vi "Set DO Status - Single.vi"(0 "reference in":refnum<class "DO.lvclass">, 2 "DO Channel Number (Zero Based)":i32, 4 "DO Status to Set":bool, 5 "error in (no error)":errorcluster) -> (14 "reference out":refnum<class "DO.lvclass">, 16 "DO Channel Number (Zero Based) OUT":i32, 19 "error out":errorcluster)   [LabVIEW 2017, in "DO.lvclass"]
uses:
  DO.lvclass
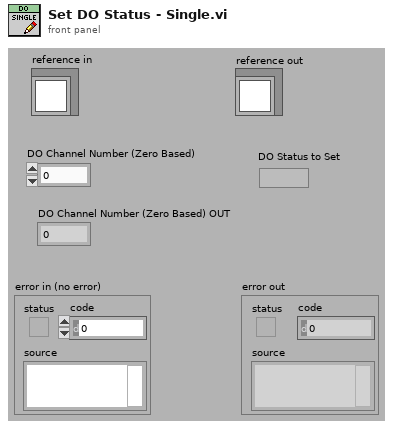
[diagram p1: front panel]
types:
  T1 = typedef "DO.lvclass/ObjectAttributes.ctl" = cluster{"DO Task":refnum<k21>, "DO Module Names (NI-Max Name)":string[], "Number of Channels Per DO Module":i32[], "DO Status":bool[], "Number of DO Modules":u32, "DO Status to Set":bool[], "DO On/Off Status":bool, "DO VI Reference":refnum<vi>, "Number of Total DO Channels":u32}
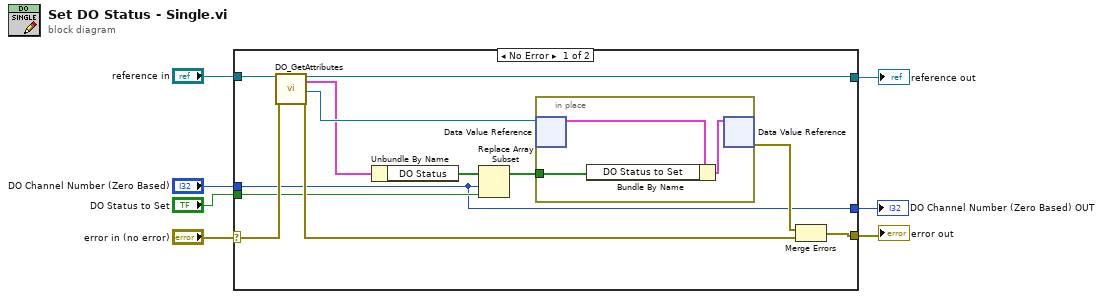
[diagram p0: block diagram]
diagram:
  n1 = case shown="No Error" "error in (no error)" {
    selector: "error in (no error)" -> [w18 w25]
    tunnel: [w15 w25] -> w6
    tunnel: [w16 w24] -> w4
    tunnel: "reference in" -> [w19 w24]
    tunnel: "DO Channel Number (Zero Based)" -> [w8 w23]
    tunnel: "DO Status to Set" -> [w11 _]
    tunnel: [w8 w23] -> w1
    frame No Error {
      n2 = call "DO_GetAttributes.vi"("reference in"=w19, "error in (no error)"=w18) -> ("reference out"=w16:refnum<class "DO.lvclass">, "Data"=w10:T1, "DataRef"=w14:refnum<data-value>, "error out"=w13:errorcluster)  [unwired: 14 in]
      n3 = Unbundle By Name(w10) -> ("DO Status"=w12:bool[])
      n4 = Replace Array Subset(array=w12, new element=w11, index=w8) -> (w9:bool[])
      n5 = in-place {
        in-place-border: w9 -> [w20]
        n6 = in-place-dvr #1(w14) -> (w22:T1)  [unwired: 1 out]
        n7 = Bundle By Name(cluster=w22, "DO Status to Set"=w20) -> (w21:T1)
        n8 = in-place-dvr #1(w21) -> (w17:errorcluster)  [unwired: 1 out]
      }
      n9 = Merge Errors(w17, w13) -> (w15:errorcluster)
    }
    frame Error {
    }
  }
  "error out" <- w6
  "reference out" <- w4
  "DO Channel Number (Zero Based) OUT" <- w1
